vi "Multiply Class Test.vi"(8 "Error In":errorcluster) -> (0 "Error Out":errorcluster)   [LabVIEW 2023, in "Test.lvlib"]
doc: "The VI is a test VI to check if the multiply class data over rides the operation method and performs multiplication properly."
uses:
  Test.lvlib
  Controls/Test Input Output.ctl
  Classes/Arithemtic Operation/Arithemetic Operation.lvclass
  <vilib>/addons/_JKI Toolkits/Caraya/classes/Assert/Assert Equal Value_Variant.vi
  <vilib>/addons/_JKI Toolkits/Caraya/classes/Test/Test.lvclass
  <vilib>/addons/_JKI Toolkits/Caraya/classes/Assert/Assert.lvclass
panel:
  # "MULTIPLY CLASS TEST"
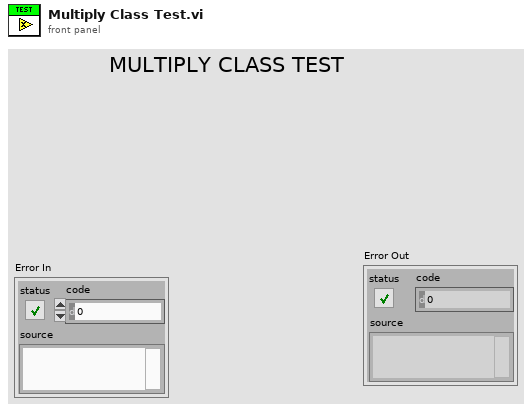
[diagram p1: front panel]
types:
  T1 = typedef "Test.lvlib/Test Input Output.ctl" = cluster{"Input 1":dbl, "Input 2":dbl, "Output":dbl}
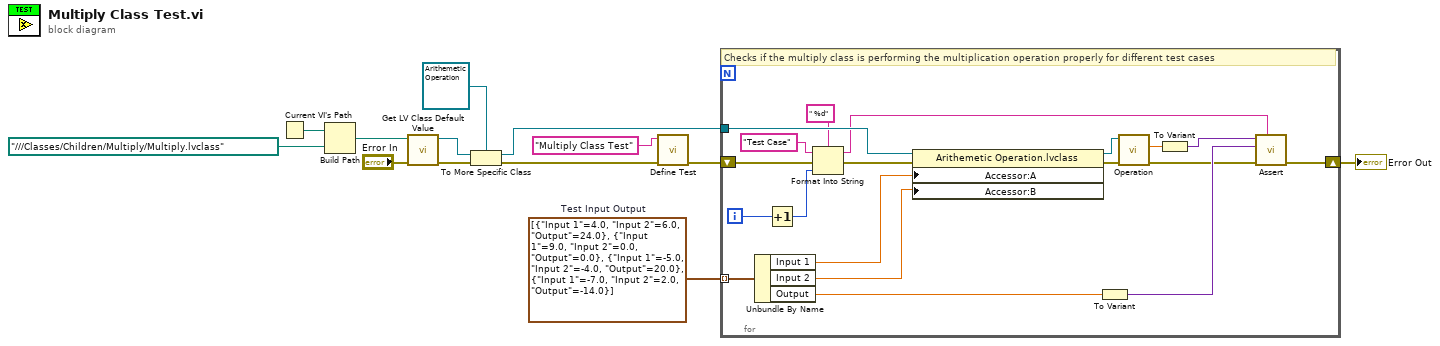
[diagram p0: block diagram]
diagram:
  w12 = T1[] [{"Input 1"=4.0, "Input 2"=6.0, "Output"=24.0}, {"Input 1"=9.0, "Input 2"=0.0, "Output"=0.0}, {"Input 1"=-5.0, "Input 2"=-4.0, "Output"=20.0}, {"Input 1"=-7.0, "Input 2"=2.0, "Output"=-14.0}]  # Test Input Output
  n1 = Current VI's Path() -> (path=w1:path)
  n2 = Build Path(base path=w1, name or relative path=path "../../../Classes/Children/Multiply/Multiply.lvclass") -> (appended path=w9:path)
  n3 = call <vilib>:"Get LV Class Default Value.vi"("error in (no error)"="Error In", "class path"=w9) -> ("error out"=w5:errorcluster, "object"=w8:refnum<class>)  [unwired: 8 in]
  n4 = To More Specific Class(target class=refnum<class "Arithemetic Operation.lvclass"> refnum ("Arithemetic Operation.lvclass"), reference=w8, error in=w5) -> (specific class reference=w6:refnum<class "Arithemetic Operation.lvclass">, error out=w4:errorcluster)
  n5 = call <vilib>:"Define Test.vi"("error in (no error)"=w4, "Label (VI Title)"="Multiply Class Test") -> ("error out"=w13:errorcluster)  [unwired: 8 in, 1 out]
  n6 = for {
    tunnel: w6 -> [w32]
    shift-right: [w30] -> w2
    shift-left: w13 -> [w31]
    tunnel: w12 -> [w29] mode=indexing
    i -> [w24]
    # "Checks if the multiply class is performing the multiplication operation properly for different test cases"
    n7 = Unbundle By Name(w29) -> ("Input 1"=w28:dbl, "Input 2"=w27:dbl, "Output"=w19:dbl)
    n8 = Increment(x=w24) -> (x+1=w23:i32)
    n9 = Format Into String(format string=" %d", initial string="Test Case", error in=w31, w23) -> (resulting string=w21:string, error out=w26:errorcluster)
    n10 = property class="Arithemetic Operation.lvclass"(reference=w32, error in=w26, "Accessor:A"=w28, "Accessor:B"=w27) -> (reference out=w14:refnum<class "Arithemetic Operation.lvclass">, error out=w17:errorcluster)
    n11 = To Variant(anything=w19) -> (Variant=w18:variant)
    n12 = call-dynamic "Operation.vi"("Error In"=w17, "Arithemetic Operation in"=w14) -> ("Error Out"=w16:errorcluster, "C"=w15:dbl)  [unwired: 7 in, 1 out]
    n13 = To Variant(anything=w15) -> (Variant=w20:variant)
    n14 = call-poly <vilib>:"Assert.vi"("Label"=w21, "error in (no error)"=w16, "Y"=w18, "X"=w20) -> ("error out"=w30:errorcluster)  [unwired: 6 in, 1 out]
  }
  "Error Out" <- w2
